vi "stoperaseCI1_tt.vi"   [LabVIEW 2013]
types:
  T1 = cluster{"CI":refnum<k21>[], "E_CI":errorcluster[]}
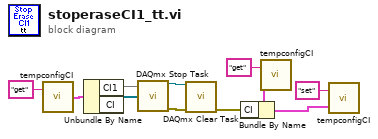
[diagram p0: block diagram]
diagram:
  n1 = call "tempconfigCI.vi"("command"="get") -> ("Temp Config out"=w8:T1)  [unwired: 1 in]
  n2 = Unbundle By Name(w8) -> ("CI1"=w7, "CI"=w6:refnum<k21>[])
  n3 = call <vilib>:"DAQmx Stop Task.vi"("task/channels in"=w7, "error in"=w6) -> ("task out"=w10:refnum<k21>, "error out"=w11:errorcluster)  [unwired: 12 in]
  n4 = call <vilib>:"DAQmx Clear Task.vi"("task in"=w10, "error in"=w11) -> ("error out"=w2:errorcluster)  [unwired: 13 in]
  n5 = call "tempconfigCI.vi"("command"="get") -> ("Temp Config out"=w3:T1)  [unwired: 1 in]
  n6 = Bundle By Name(cluster=w3, "CI"=w2) -> (w1:T1)
  n7 = call "tempconfigCI.vi"("Temp Config in"=w1, "command"="set") -> ()  [unwired: 1 out]
